vi "PutInt16.vi"(8 "error in (no error)":errorcluster, 10 "Number":i16, 11 "MsgPackSerializer in":refnum<class "MsgPackSerializer.lvclass">) -> (0 "error out":errorcluster, 3 "MsgPackSerializer out":refnum<class "MsgPackSerializer.lvclass">)   [LabVIEW 2015, in "MsgPackSerializer.lvclass"]
uses:
  MsgPackSerializer.lvclass
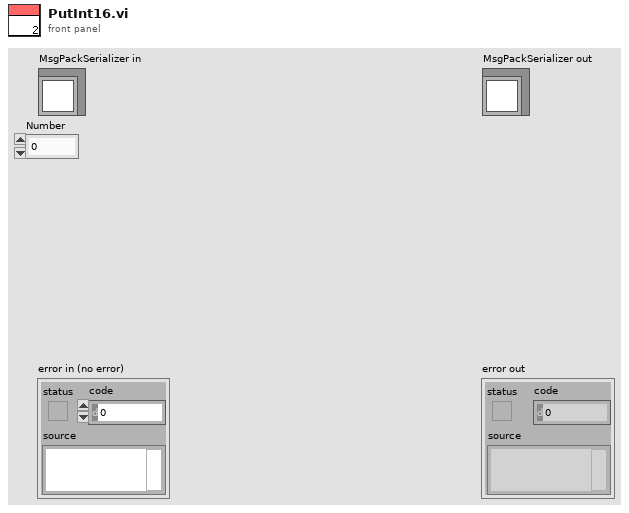
[diagram p1: front panel]
types:
  T1 = enum16{"big-endian, network order", "native, host order", "little-endian"}
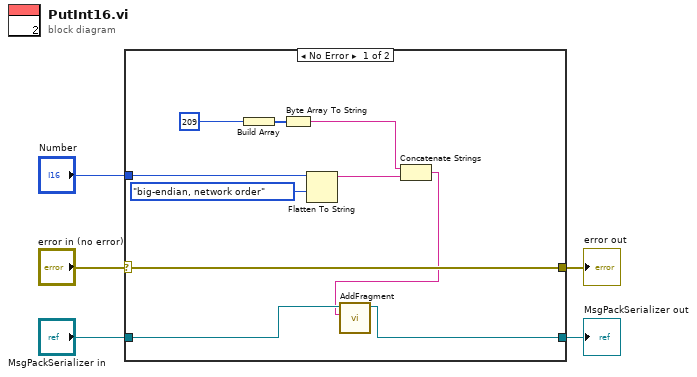
[diagram p0: block diagram]
diagram:
  n1 = case shown="No Error" "error in (no error)" {
    selector: "error in (no error)" -> [w15 w17]
    tunnel: [w15 w17] -> w4
    tunnel: [w11 w16] -> w2
    tunnel: "MsgPackSerializer in" -> [w12 w16]
    tunnel: "Number" -> [w14 _]
    frame No Error {
      n2 = Build Array(u8 209 ("Number")) -> (w10:u8[])
      n3 = Byte Array To String(unsigned byte array=w10) -> (string=w7:string)
      n4 = Flatten To String(anything=w14, byte order (0:big-endian, network order)=T1."big-endian, network order") -> (data string=w8:string)  [unwired: 2 in, 2 out]
      n5 = Concatenate Strings(w7, w8) -> (w6:string)
      n6 = call "AddFragment.vi"("Fragment"=w6, "MsgPackSerializer in"=w12) -> ("MsgPackSerializer out"=w11:refnum<class "MsgPackSerializer.lvclass">)  [unwired: 8 in, 1 out]
    }
    frame Error {
    }
  }
  "error out" <- w4
  "MsgPackSerializer out" <- w2
